vi "CleanCompleteFFTArray.vi"(8 "Complete FFT Array":dbl[](array[numeric]), 10 "FFT Size":i32=512, 11 "#Signals":i32=1) -> (0 "Second Edge Array":dbl[](array[numeric]), 3 "First Edge Array":dbl[](array[numeric]))   [LabVIEW 2014]
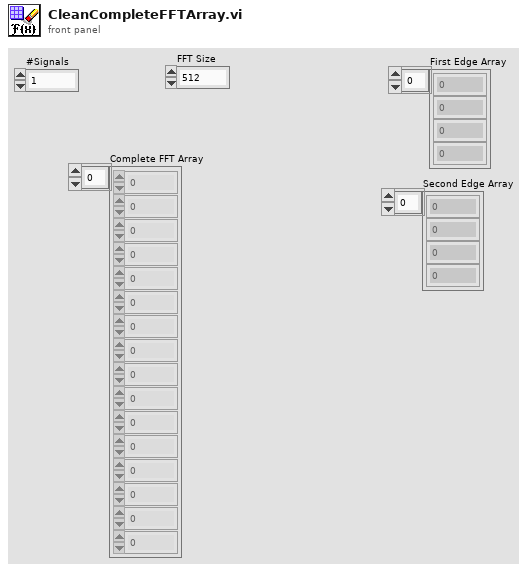
[diagram p1: front panel]
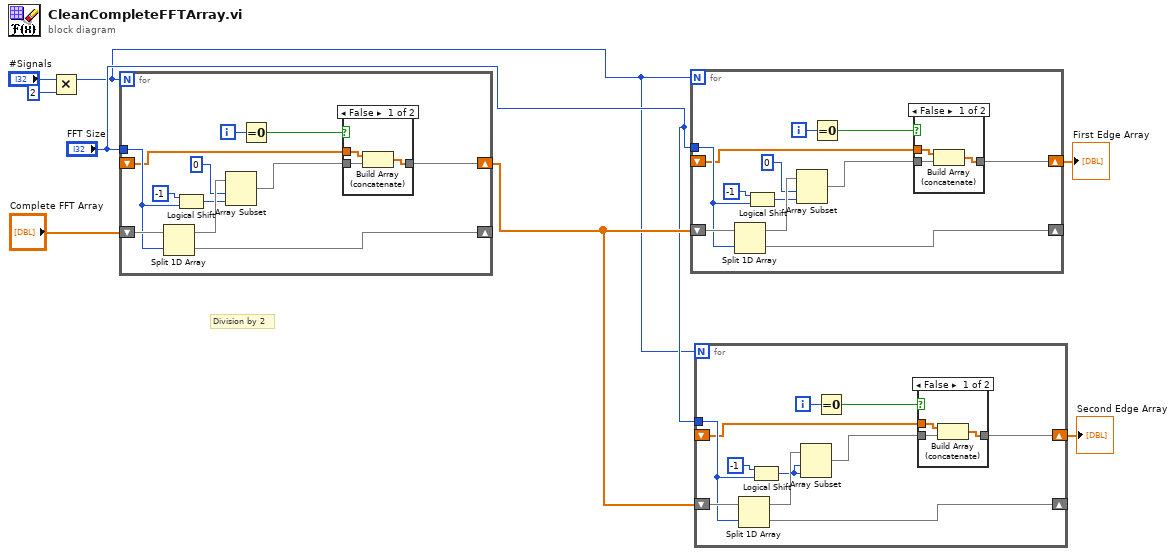
[diagram p0: block diagram]
diagram:
  # "Division by 2"
  n1 = Multiply(x="#Signals", y=2) -> (x*y=w2:i32)
  n2 = for {
    N: w2 -> [_]
    shift-right: [w19] -> _
    shift-left: "Complete FFT Array" -> [w20]
    tunnel: "FFT Size" -> [w14]
    shift-right: [w9] -> w7
    shift-left: _ -> [w10]
    i -> [w16]
    n3 = Split 1D Array(array=w20, index=w14) -> (first subarray=w18:dbl[], second subarray=w19:dbl[])
    n4 = Logical Shift(y=i16 -1, x=w14) -> (x << y=w12:i32)
    n5 = Array Subset(array=w18, index=0, length=w12) -> (w11:dbl[])
    n6 = Equal To 0?(x=w16) -> (x = 0?=w15:bool)
    n7 = case shown="False" w15 {
      tunnel: w11 -> [w23 w24]
      tunnel: w10 -> [w22 _]
      tunnel: [w21 w24] -> w9
      frame False {
        n8 = Build Array (concatenate)(w22, w23) -> (w21:dbl[])
      }
      frame True {
      }
    }
  }
  n9 = for {
    N: w2 -> [_]
    shift-right: [w35] -> _
    shift-left: w7 -> [w36]
    tunnel: "FFT Size" -> [w30]
    shift-right: [w25] -> w4
    shift-left: _ -> [w26]
    i -> [w32]
    n10 = Split 1D Array(array=w36, index=w30) -> (first subarray=w34:dbl[], second subarray=w35:dbl[])
    n11 = Logical Shift(y=i16 -1, x=w30) -> (x << y=w28:i32)
    n12 = Array Subset(array=w34, index=0, length=w28) -> (w27:dbl[])
    n13 = Equal To 0?(x=w32) -> (x = 0?=w31:bool)
    n14 = case shown="False" w31 {
      tunnel: w27 -> [w39 w40]
      tunnel: w26 -> [w38 _]
      tunnel: [w37 w40] -> w25
      frame False {
        n15 = Build Array (concatenate)(w38, w39) -> (w37:dbl[])
      }
      frame True {
      }
    }
  }
  "First Edge Array" <- w4
  n16 = for {
    N: w2 -> [_]
    shift-right: [w50] -> _
    shift-left: w7 -> [w51]
    tunnel: "FFT Size" -> [w46]
    shift-right: [w42] -> w3
    shift-left: _ -> [w43]
    i -> [w48]
    n17 = Split 1D Array(array=w51, index=w46) -> (first subarray=w49:dbl[], second subarray=w50:dbl[])
    n18 = Logical Shift(y=i16 -1, x=w46) -> (x << y=w41:i32)
    n19 = Array Subset(array=w49, index=w41, length=w41) -> (w44:dbl[])
    n20 = Equal To 0?(x=w48) -> (x = 0?=w47:bool)
    n21 = case shown="False" w47 {
      tunnel: w44 -> [w54 w55]
      tunnel: w43 -> [w53 _]
      tunnel: [w52 w55] -> w42
      frame False {
        n22 = Build Array (concatenate)(w53, w54) -> (w52:dbl[])
      }
      frame True {
      }
    }
  }
  "Second Edge Array" <- w3
